vi "start_sweep.vi"(8 "error in (no error)":errorcluster, 11 "DL090430TriggeredExperimentController in":refnum<class "ExperimentControllerDL090430DAQmxTriggered.lvclass">) -> (0 "error out":errorcluster, 3 "DL090430TriggeredExperimentController out":refnum<class "ExperimentControllerDL090430DAQmxTriggered.lvclass">)   [LabVIEW 2010, in "ExperimentControllerDL090430DAQmxTriggered.lvclass"]
uses:
  ExperimentControllerDL090430DAQmxTriggered.lvclass
  ExperimentControllerDL090430DAQmxTriggered.lvclass/ExperimentControllerDL090430DAQmxTriggered.ctl
  ImagingMode/GenericImagingMode/GenericImagingMode/GenericImagingMode.lvclass
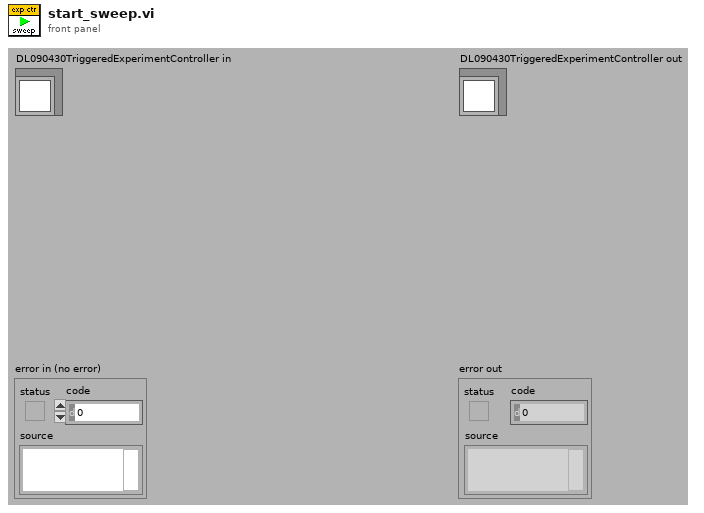
[diagram p1: front panel]
types:
  T1 = typedef "GenericToplevelComponent.lvclass/common_trigger_enum.ctl" = enum16{"NULL", "initialise", "terminate", "fetch command", "fetch data", "attach observer", "register as observer", "detach observer", "acknowledge", "start", "stop", "sweep started", "sweep finished", "experiment started", "experiment stopped"}
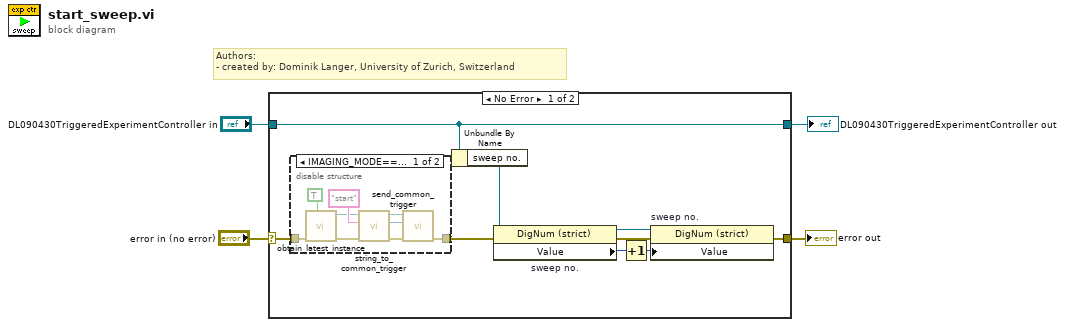
[diagram p0: block diagram]
diagram:
  # "Authors: \n- created by: Dominik Langer, University of Zurich, Switzerland"
  n1 = case shown="No Error" "error in (no error)" {
    selector: "error in (no error)" -> [w6 w25]
    tunnel: [w9 w25] -> w3
    tunnel: [w13 w24] -> w1
    tunnel: "DL090430TriggeredExperimentController in" -> [w13 w24]
    frame No Error {
      n2 = disable-structure shown="IMAGING_MODE==1" {
        disable-tunnel: w6 -> [w22 w23]
        disable-tunnel: [w21 w23] -> w5
        frame condition #0 {
          n3 = call "obtain_latest_instance.vi"("quick, but maybe outdated?"=TRUE, "error in (no error)"=w22) -> ("error out"=w18:errorcluster, "GenericScanMode out"=w17:refnum<class "GenericImagingMode.lvclass">)  [unwired: 8 in]
          n4 = call-dynamic "string_to_common_trigger.vi"("error in (no error)"=w18, "trigger string"="start", "GenericToplevelComponent in"=w17) -> ("error out"=w16:errorcluster, "trigger"=w15:T1, "GenericToplevelComponent out"=w14:refnum<class "GenericImagingMode.lvclass">)  [unwired: 6 in]
          n5 = call-dynamic "send_common_trigger.vi"("error in (no error)"=w16, "trigger"=w15, "GenericToplevelComponent in"=w14) -> ("error out"=w21:errorcluster)  [unwired: 6 in, 2 out]
        }
        frame condition #1 (active) {
        }
      }
      n6 = Unbundle By Name(w13) -> ("sweep no."=w12:refnum<vi>)
      n7 = property on="sweep no." class="DigNum (strict)"(reference=w12, error in=w5) -> (reference out=w10:refnum<vi>, error out=w11:errorcluster, "Value"=w8:i32)
      n8 = Increment(x=w8) -> (x+1=w7:i32)
      n9 = property on="sweep no." class="DigNum (strict)"(reference=w10, error in=w11, "Value"=w7) -> (error out=w9:errorcluster)  [unwired: 1 out]
    }
    frame Error {
    }
  }
  "error out" <- w3
  "DL090430TriggeredExperimentController out" <- w1
